vi "FlipArray2.vi"() -> ()   [LabVIEW 2018]
panel:
  out "Array":dbl[](array[numeric])
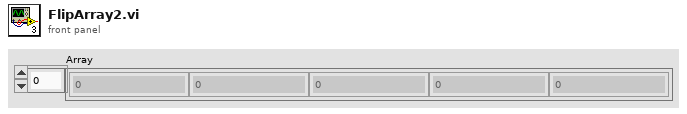
[diagram p1: front panel]
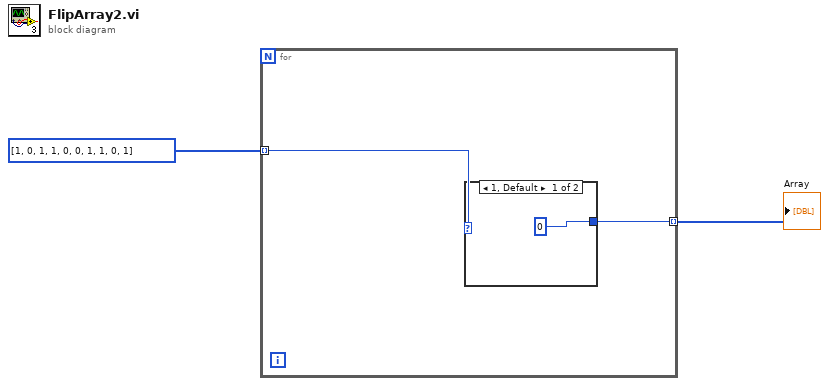
[diagram p0: block diagram]
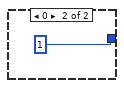
[diagram p2: hidden frame]
diagram:
  n1 = for {
    tunnel: i32[] [1, 0, 1, 1, 0, 0, 1, 1, 0, 1] -> [w4] mode=indexing
    tunnel: [w3] -> w1 mode=indexing
    n2 = case shown="1, Default" w4 {
      tunnel: [0 1] -> w3
      frame 1, Default {
      }
      frame 0 {
      }
    }
  }
  "Array" <- w1
